vi "Set Flight Mode.vi"(8 "Error In":errorcluster) -> (0 "Error Out":errorcluster)   [LabVIEW 2014]
uses:
  <vilib>/Platform/TimedLoop/XDataNode/timing_clust.ctl
  <vilib>/Platform/TimedLoop/XDataNode/nitl_modes.ctl
  <vilib>/Platform/TimedLoop/XDataNode/wakeup.ctl
  MAVLink/Controls/MAVLink Flight modes.ctl
  Web Services/DronePi Global Variables.vi
  <vilib>/platform/TimedLoop/XDataNode/XDataNode.xnode
  <vilib>/Platform/TimedLoop/XDataNode/XDNodeRunTimeDep.lvlib
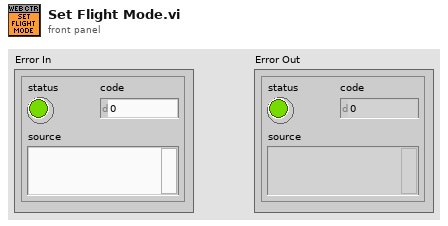
[diagram p1: front panel]
types:
  T1 = typedef "XDNodeRunTimeDep.lvlib/timing_clust.ctl" = cluster{"Expected End [f-1]":u64, "Actual End [f-1]":u64, "Finished Late? [f-1]":bool, "Expected End [i-1]":u64, "Actual End [i-1]":u64, "Finished Late? [i-1]":bool, "Expected Start [i]":u64, "Actual Start [i]":u64, "Expected Start [f]":u64, "Actual Start [f]":u64, "Source Name":string, "Structure Name":string, "Period":i64, "Deadline":i64, "Offset":i64, "Start":i64, "Priority":i32, "Timeout":i32, "Mode":T2, "Wakeup Reason":T3, "Error":errorcluster, "Source Type":string, "Secondary Source Type":string, "Global End Time":u64, "Global Start Time":u64, "Frame Duration":u64, "Iteration Duration":u64, "Assigned CPU":i32, "I/O Scan Engine Mode":u32}
  T2 = typedef "XDNodeRunTimeDep.lvlib/nitl_modes.ctl" = enum32{"No Change", "Process missed periods, maintain original phase", "Discard missed periods, maintain original phase", "Process missed periods, ignore original phase", "Discard missed periods, ignore original phase"}
  T3 = typedef "XDNodeRunTimeDep.lvlib/wakeup.ctl" = enum32{"Normal", "Aborted", "Asynchronous wakeup", "Timing source error", "Timed loop error", "Timeout"}
  T4 = typedef "MAVLink Flight modes.ctl" = enum32{"STABILISE", "ACRO", "ALT HOLD", "AUTO", "GUIDED", "LOITER", "RTL", "CIRCLE", "UNKNOWN1", "LAND", "OF LOITER", "DRIFT", "UNKNOWN2", "SPORT", "FLIP", "AUTO TUNE", "POS HOLD", "BRAKE"}
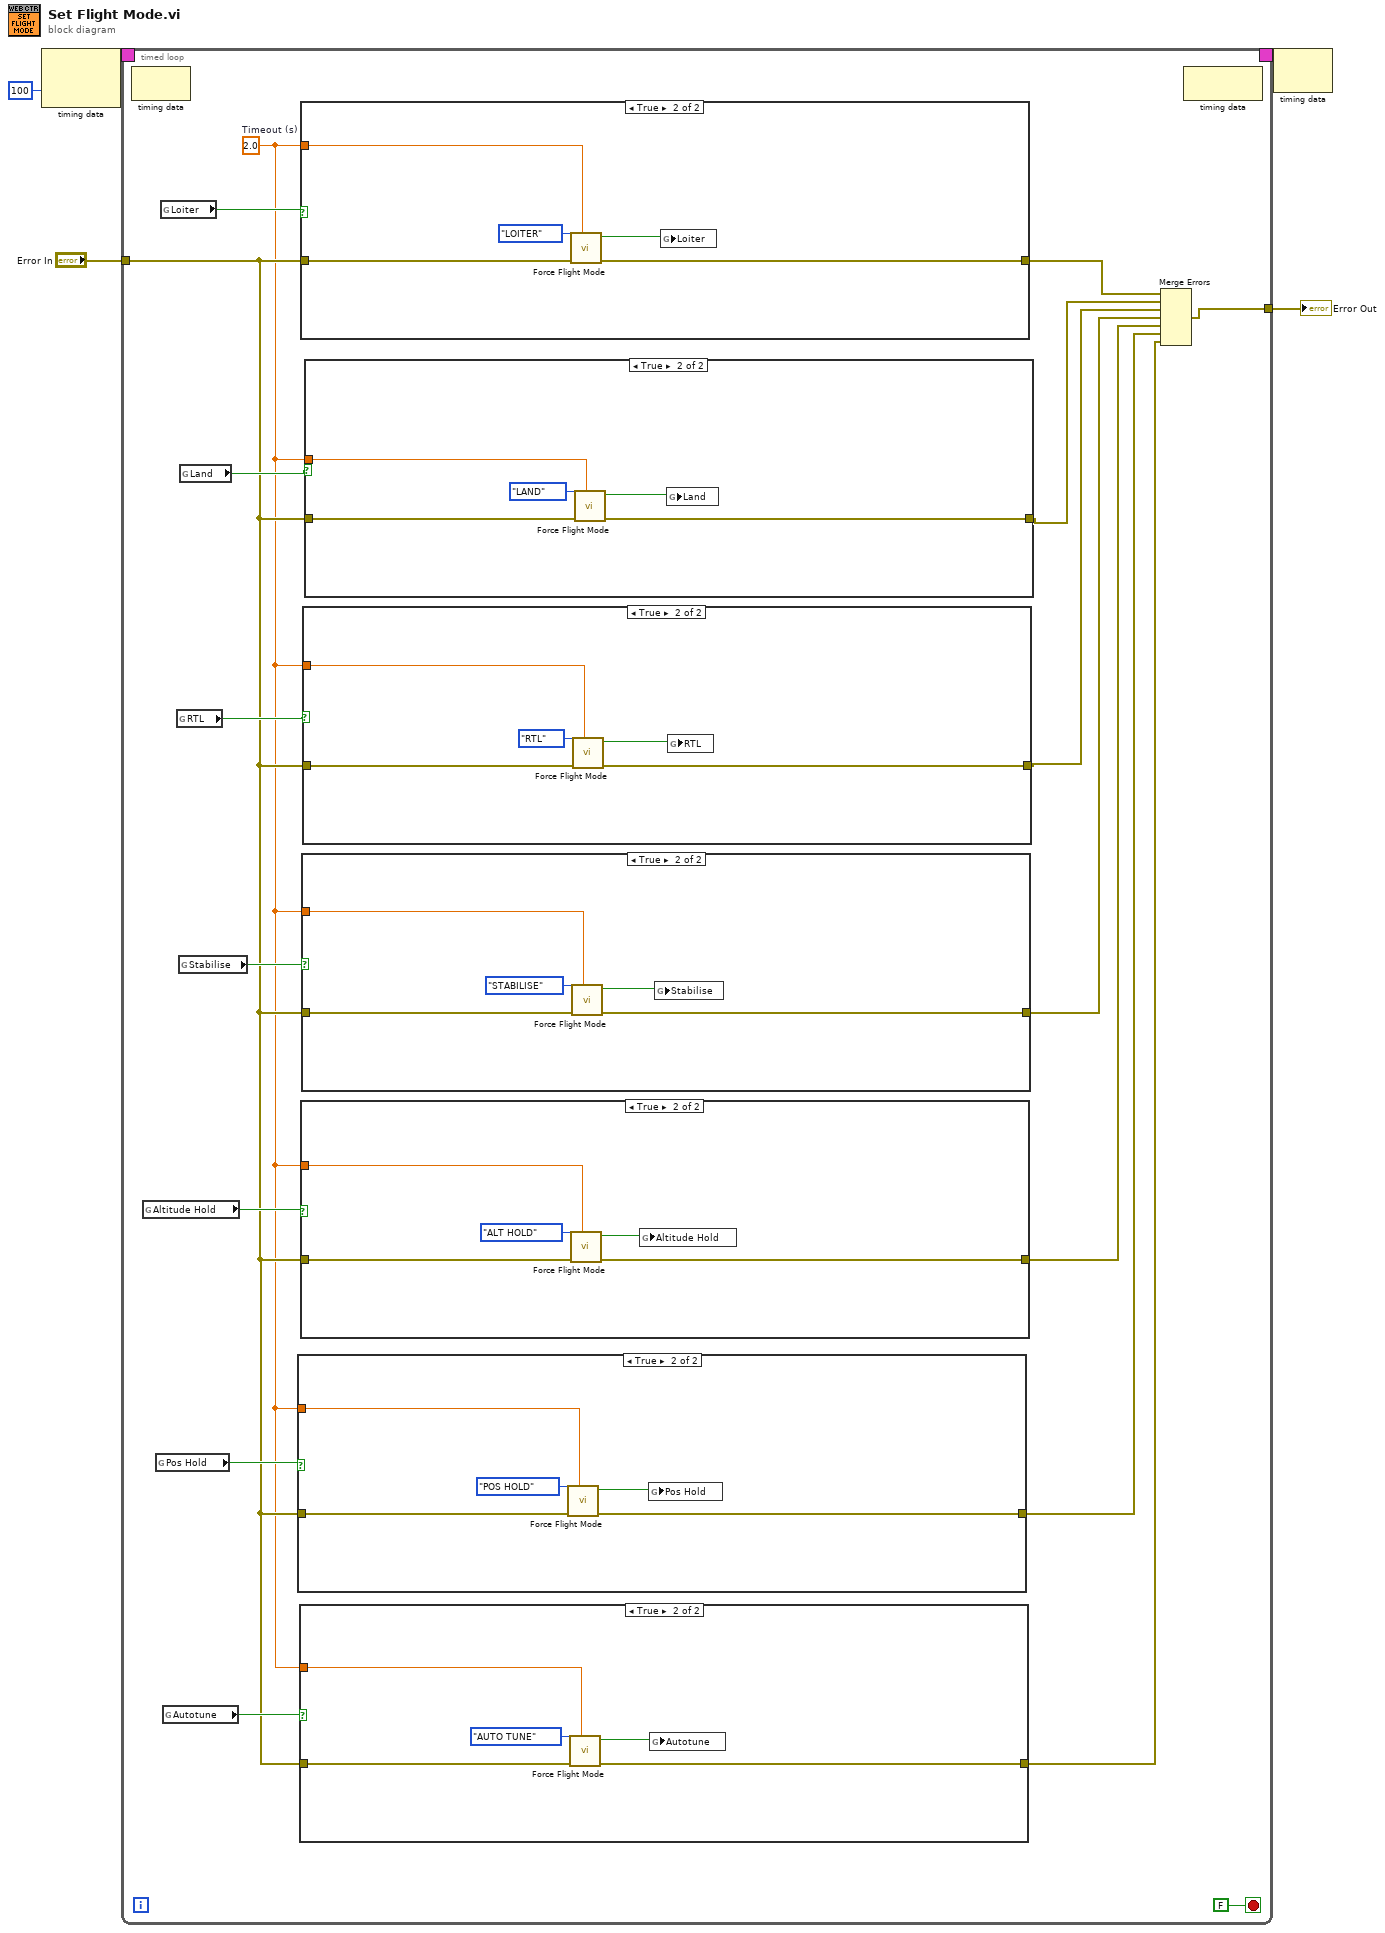
[diagram p0: block diagram]
diagram:
  n1 = node-c288(i64 100 ("Period")) -> (w5:T1)  [unwired: 1 in]
  n2 = timed-loop {
    timing: w5 -> [_]
    timing-out: [_] -> w4
    tunnel: [w8] -> w3
    tunnel: "Error In" -> [w7]
    stop <- FALSE stop-if-true
    w6 = 2.0  # Timeout (s)
    n3 = node-c288() -> ()  [unwired: 1 in, 1 out]
    n4 = global read "DronePi Global Variables.vi" "Altitude Hold"() -> (w13:bool)
    n5 = global read "DronePi Global Variables.vi" "Pos Hold"() -> (w12:bool)
    n6 = global read "DronePi Global Variables.vi" "Loiter"() -> (w23:bool)
    n7 = global read "DronePi Global Variables.vi" "Autotune"() -> (w11:bool)
    n8 = global read "DronePi Global Variables.vi" "RTL"() -> (w20:bool)
    n9 = global read "DronePi Global Variables.vi" "Stabilise"() -> (w14:bool)
    n10 = global read "DronePi Global Variables.vi" "Land"() -> (w21:bool)
    n11 = case shown="True" w12 {
      tunnel: w7 -> [w30 w34]
      tunnel: [w30 w32] -> w15
      tunnel: w6 -> [_ w31]
      frame False {
      }
      frame True {
        n12 = call "Force Flight Mode.vi"("Timeout (s)"=w31, "Error In"=w34, "Aircraft Mode"=MAVLink_Flight_modes."POS HOLD") -> ("Error Out"=w32:errorcluster, "reset button state"=w33:bool)  [unwired: 7 in]
        n13 = global write "DronePi Global Variables.vi" "Pos Hold"(w33) -> ()
      }
    }
    n14 = case shown="True" w11 {
      tunnel: w7 -> [w24 w28]
      tunnel: [w24 w26] -> w10
      tunnel: w6 -> [_ w25]
      frame False {
      }
      frame True {
        n15 = call "Force Flight Mode.vi"("Timeout (s)"=w25, "Error In"=w28, "Aircraft Mode"=MAVLink_Flight_modes."AUTO TUNE") -> ("Error Out"=w26:errorcluster, "reset button state"=w27:bool)  [unwired: 7 in]
        n16 = global write "DronePi Global Variables.vi" "Autotune"(w27) -> ()
      }
    }
    n17 = case shown="True" w23 {
      tunnel: w7 -> [w60 w64]
      tunnel: [w60 w62] -> w22
      tunnel: w6 -> [_ w61]
      frame False {
      }
      frame True {
        n18 = call "Force Flight Mode.vi"("Timeout (s)"=w61, "Error In"=w64, "Aircraft Mode"=MAVLink_Flight_modes."LOITER") -> ("Error Out"=w62:errorcluster, "reset button state"=w63:bool)  [unwired: 7 in]
        n19 = global write "DronePi Global Variables.vi" "Loiter"(w63) -> ()
      }
    }
    n20 = case shown="True" w13 {
      tunnel: w7 -> [w36 w40]
      tunnel: [w36 w38] -> w16
      tunnel: w6 -> [_ w37]
      frame False {
      }
      frame True {
        n21 = call "Force Flight Mode.vi"("Timeout (s)"=w37, "Error In"=w40, "Aircraft Mode"=MAVLink_Flight_modes."ALT HOLD") -> ("Error Out"=w38:errorcluster, "reset button state"=w39:bool)  [unwired: 7 in]
        n22 = global write "DronePi Global Variables.vi" "Altitude Hold"(w39) -> ()
      }
    }
    n23 = case shown="True" w14 {
      tunnel: w7 -> [w42 w46]
      tunnel: [w42 w44] -> w17
      tunnel: w6 -> [_ w43]
      frame False {
      }
      frame True {
        n24 = call "Force Flight Mode.vi"("Timeout (s)"=w43, "Error In"=w46, "Aircraft Mode"=MAVLink_Flight_modes."STABILISE") -> ("Error Out"=w44:errorcluster, "reset button state"=w45:bool)  [unwired: 7 in]
        n25 = global write "DronePi Global Variables.vi" "Stabilise"(w45) -> ()
      }
    }
    n26 = case shown="True" w20 {
      tunnel: w7 -> [w48 w52]
      tunnel: [w48 w50] -> w18
      tunnel: w6 -> [_ w49]
      frame False {
      }
      frame True {
        n27 = call "Force Flight Mode.vi"("Timeout (s)"=w49, "Error In"=w52, "Aircraft Mode"=MAVLink_Flight_modes."RTL") -> ("Error Out"=w50:errorcluster, "reset button state"=w51:bool)  [unwired: 7 in]
        n28 = global write "DronePi Global Variables.vi" "RTL"(w51) -> ()
      }
    }
    n29 = case shown="True" w21 {
      tunnel: w7 -> [w54 w58]
      tunnel: [w54 w56] -> w19
      tunnel: w6 -> [_ w55]
      frame False {
      }
      frame True {
        n30 = call "Force Flight Mode.vi"("Timeout (s)"=w55, "Error In"=w58, "Aircraft Mode"=MAVLink_Flight_modes."LAND") -> ("Error Out"=w56:errorcluster, "reset button state"=w57:bool)  [unwired: 7 in]
        n31 = global write "DronePi Global Variables.vi" "Land"(w57) -> ()
      }
    }
    n32 = Merge Errors(w22, w19, w18, w17, w16, w15, w10) -> (w8:errorcluster)
    n33 = node-c288() -> ()  [unwired: 1 in, 1 out]
  }
  "Error Out" <- w3
  n34 = node-c288(w4) -> ()  [unwired: 1 out]
